vi "Actor Core.vi"(8 "error in":errorcluster, 11 "Caller in":refnum<class "Nested.lvclass">) -> (0 "error out":errorcluster, 3 "Actor out":refnum<class "Actor.lvclass">)   [LabVIEW 2020, in "Nested.lvlib" / "Nested.lvclass"]
doc: "(<B>Filename</B>: Actor Framework.lvlib:Actor.lvclass:Actor Core.vi)\n\nReceives messages to the actor, reacts to them, and initiates any error handling that may shut the actor down.\n\nDescendant classes may override this VI to append parallel tasks for the actor to complete while it handles messages. Overrides use the Call Parent Class Method node."
uses:
  Nested.lvclass
  <vilib>/ActorFramework/Actor/Actor.lvclass
  Nested.lvclass/Nested.ctl
  Nested Messages/UpdateDIsplayNested Msg/UpdateDIsplayNested Msg.lvclass/UpdateDIsplayNested Msg.ctl
  <vilib>/ActorFramework/Message Enqueuer/Message Enqueuer.lvclass/Message Enqueuer.ctl
  <vilib>/ActorFramework/Message Enqueuer/Enqueue.vi
  Nested Messages/UpdateDIsplayNested Msg/UpdateDIsplayNested Msg.lvclass
  C:/Program Files/National Instruments/LabVIEW 2020/vi.lib/ActorFramework/Message/Message.lvclass
  Nested Messages/Error Msg/Error Msg.lvclass
  <vilib>/ActorFramework/Stop Msg/Stop Msg.lvclass
  <vilib>/ActorFramework/Message Priority Queue/Priority Enqueue.vi
panel:
  in  "Btn_Error":bool
  in  "Message":string
  out "Display":string
  in  "Btn_ Sendmsg_Caller":bool
  # "Nested"
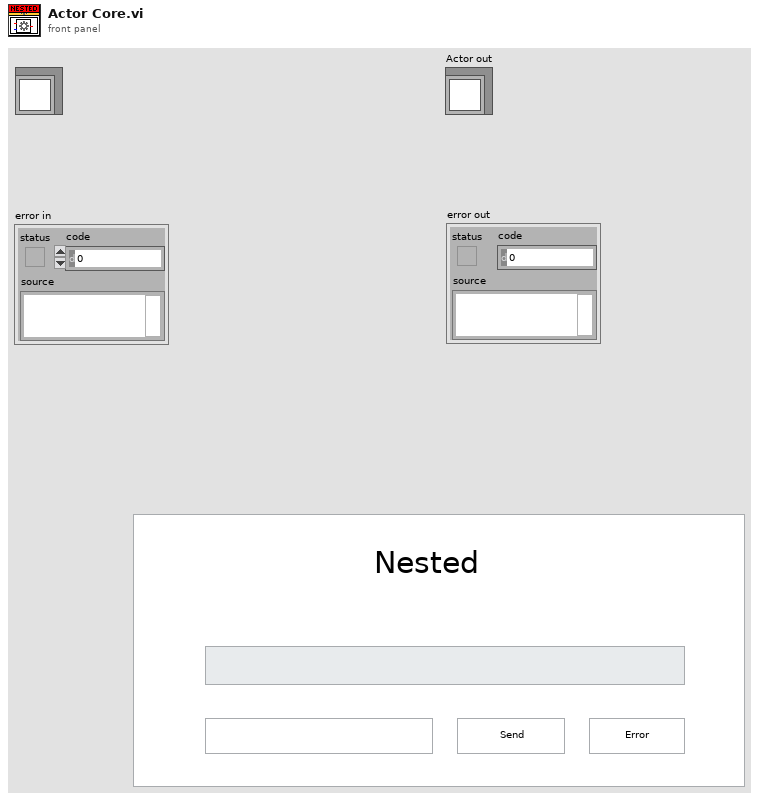
[diagram p1: front panel]
types:
  T1 = cluster{"Quit":refnum<user-event>, "Update Display":refnum<user-event>}
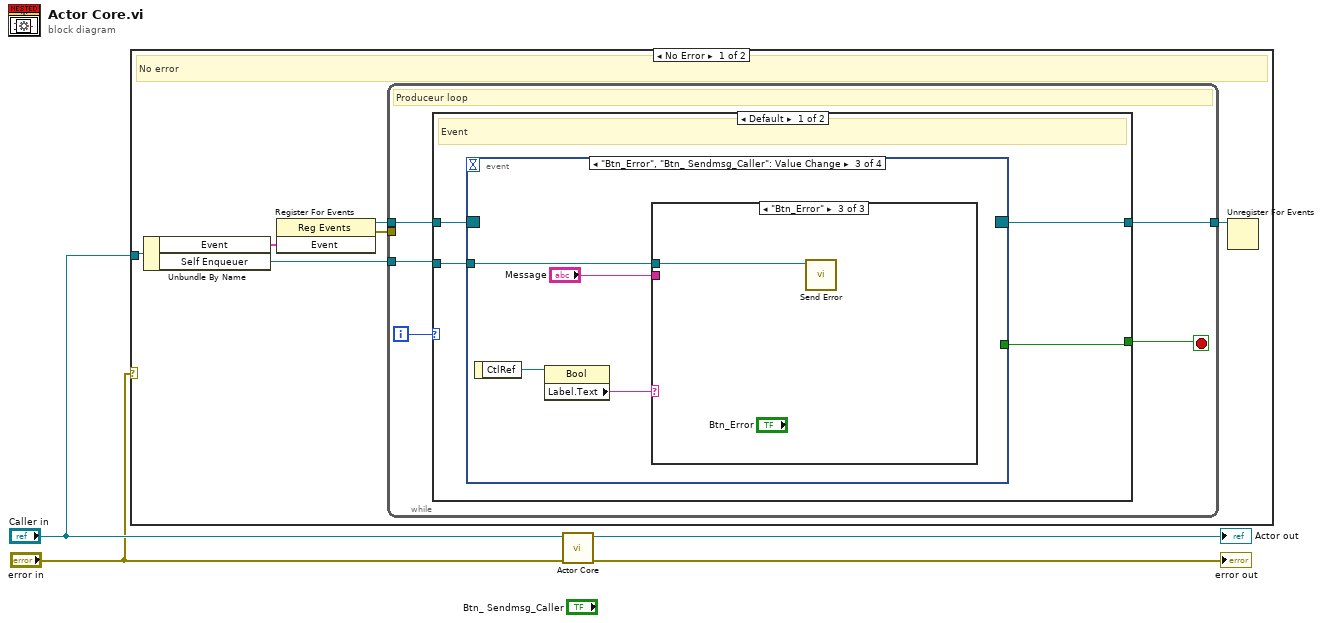
[diagram p0: block diagram]
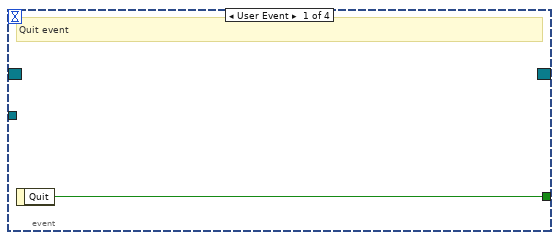
[diagram p2: hidden frame]
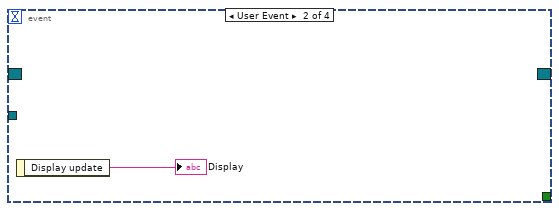
[diagram p3: hidden frame]
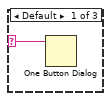
[diagram p4: hidden frame]
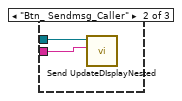
[diagram p5: hidden frame]
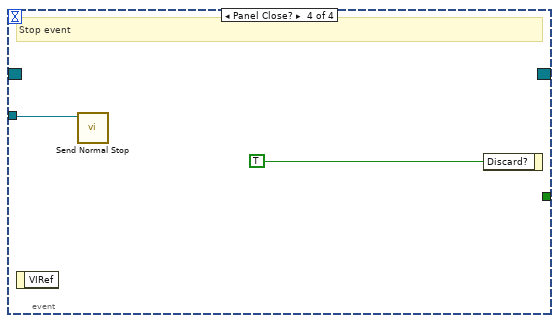
[diagram p6: hidden frame]
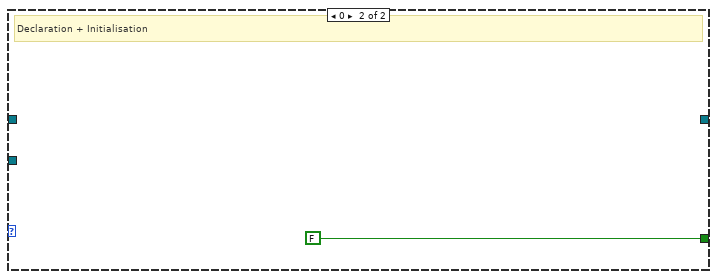
[diagram p7: hidden frame]
diagram:
  n1 = case shown="No Error" "error in" {
    tunnel: "Caller in" -> [w8 _]
    frame No Error {
      # "No error"
      n2 = Unbundle By Name(w8) -> ("Event"=w6:T1, "Self Enqueuer"=w9:refnum<class "Message Enqueuer.lvclass">)
      n3 = register-events(w6) -> (reference out=w7:refnum<event-registration>, error out=w5:errorcluster)  [unwired: 2 in]
      n4 = while {
        tunnel: [w13] -> w10
        tunnel: w9 -> [w12]
        tunnel: w7 -> [w11]
        tunnel: w5 -> [_]
        i -> [w15]
        stop <- w14 stop-if-true
        # "Produceur loop"
        n5 = case shown="Default" w15 {
          tunnel: w12 -> [w17 _]
          tunnel: [w18 FALSE] -> w14
          tunnel: [w19 _] -> w13
          tunnel: w11 -> [w16 _]
          frame Default {
            # "Event"
            n6 = event shown="[2] \"Btn_Error\", \"Btn_ Sendmsg_Caller\": Value Change" {
              selector: w16 -> [_ _ _ _]
              dyn-events: [_ _ _ _] -> w19
              timeout: _ -> [_ _ _ _]
              tunnel: [w20 _ _ _] -> w18
              tunnel: w17 -> [_ _ w23 w30]
              event User Event {
                # "Quit event"
                n7 = event-data() -> ("Quit"=w20:bool)  [unwired: 1 in]
              }
              event User Event {
                n8 = event-data() -> ("Display update"=→"Display":string)  [unwired: 1 in]
              }
              event "Btn_Error", "Btn_ Sendmsg_Caller": Value Change {
                n9 = event-data() -> ("CtlRef"=w25:refnum<vi>)  [unwired: 1 in]
                n10 = property class="Bool"(reference=w25) -> ("Label.Text"=w24:string)  [unwired: 1 in, 2 out]
                n11 = case shown="\"Btn_Error\"" w24 {
                  selector: w24 -> [w26 _ _]
                  tunnel: w23 -> [_ w28 w29]
                  tunnel: "Message" -> [_ w27 _]
                  frame Default {
                    n12 = One Button Dialog(message=w26) -> ()  [unwired: 1 in, 1 out]
                  }
                  frame "Btn_ Sendmsg_Caller" {
                    n13 = call "Send UpdateDIsplayNested.vi"("Message"=w27, "Message Enqueuer"=w28) -> ()  [unwired: 8 in, 2 out]
                  }
                  frame "Btn_Error" {
                    n14 = call "Send Error.vi"("Message Enqueuer"=w29) -> ()  [unwired: 9 in, 2 out]
                  }
                }
              }
              event Panel Close? {
                # "Stop event"
                n15 = event-data() -> ()  [unwired: 1 in, 1 out]
                n16 = call <vilib>:"Send Normal Stop.vi"("Message Enqueuer"=w30) -> ()  [unwired: 10 in, 1 out]
                n17 = event-data("Discard?"=TRUE) -> ()  [unwired: 1 in, 1 out]
              }
            }
          }
          frame 0 {
            # "Declaration + Initialisation"
          }
        }
      }
      n18 = Unregister For Events(event registration refnum=w10) -> ()  [unwired: 1 in, 1 out]
    }
    frame Error {
    }
  }
  n19 = call-parent "Actor Core.vi"("error in"="error in", "Actor in"="Caller in") -> ("error out"=→"error out":errorcluster, "Actor out"=→"Actor out":refnum<class "Actor.lvclass">)  [unwired: 8 in]
